vi "Open Audio File Read (Core).vi"(8 "error in (no error)":errorcluster, 11 "Path":string) -> (0 "error out":errorcluster, 3 "Audio File Refnum":T1)   [LabVIEW 2020, in "G-Audio.lvlib"]
doc: "Opens an audio file and initializes the relevant decoder.\n\nSupported codecs: flac, mp3, vorbis (ogg), and wav."
uses:
  G-Audio.lvlib
  <vilib>/Utility/error.llb/Error Cluster From Error Code.vi
  lib/g_audio_32.dll
  Controls/Audio File Refnum.ctl
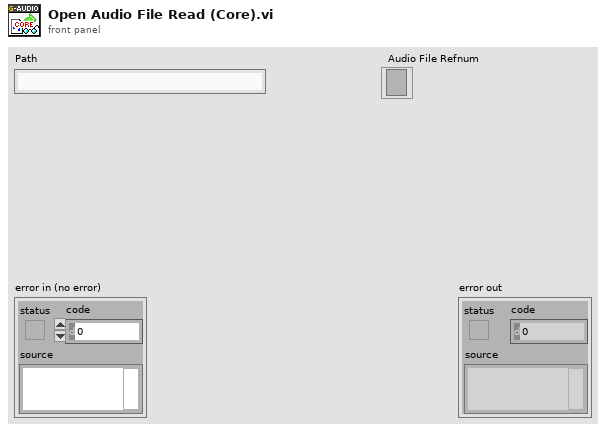
[diagram p1: front panel]
types:
  T1 = typedef "G-Audio.lvlib/Audio File Refnum.ctl" = refnum<file>
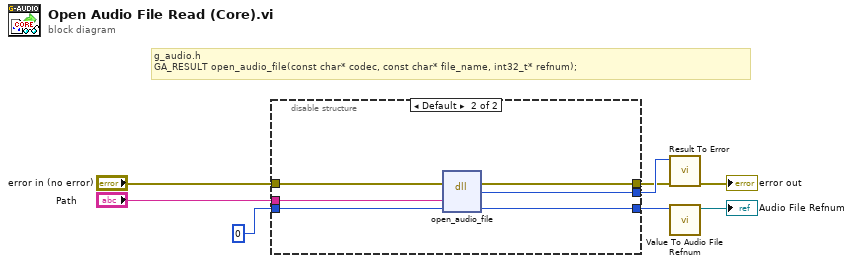
[diagram p0: block diagram]
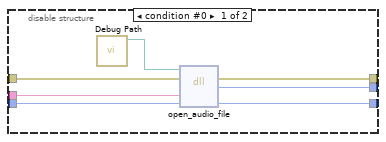
[diagram p2: hidden frame]
diagram:
  # "g_audio.h\nGA_RESULT open_audio_file(const char* codec, const char* file_name, int32_t* refnum);"
  n1 = disable-structure shown="Default" {
    disable-tunnel: "error in (no error)" -> [w15 w21]
    disable-tunnel: "Path" -> [w13 w19]
    disable-tunnel: [w14 w20] -> w5
    disable-tunnel: 0 ("num_samples") -> [w12 w18]
    disable-tunnel: [w11 w17] -> w1
    disable-tunnel: [w10 w16] -> w6
    frame condition #0 {
      n2 = call "Debug Path.vi"() -> ("Debug Path"=w9:path)  [unwired: 11 in]
      n3 = dll-call lib="?" fn="open_audio_file"(path in=w9, error in=w15, "file_name"=w13, "refnum"=w12) -> (error out=w14:errorcluster, "result"=w10:i32, "refnum"=w11:i32)  [unwired: 2 in, 1 out]
    }
    frame condition #1 (active) {
      n4 = dll-call lib="C:/github/dataflowg/g-audio/src/LabVIEW/G-Audio/lib/g_audio_*.*" fn="open_audio_file"(error in=w21, "file_name"=w19, "refnum"=w18) -> (error out=w20:errorcluster, "result"=w16:i32, "refnum"=w17:i32)  [unwired: 3 in, 1 out]
    }
  }
  n5 = call "Result To Error.vi"("error in (no error)"=w5, "Result Code"=w6) -> ("error out"=→"error out":errorcluster)  [unwired: 9 in]
  n6 = call "Value To Audio File Refnum.vi"("Refnum Value"=w1) -> ("Audio File Refnum"=→"Audio File Refnum":T1)  [unwired: 10 in]
